vi "分析光源均勻度.vi"(7 "ShowData":bool, 8 "error in (no error)":errorcluster, 10 "DieArea":i32 min=10, 11 "Image In":T1) -> (0 "error out":errorcluster, 3 "Image":T1)   [LabVIEW 2015]
uses:
  <vilib>/vision/Image Controls.llb/IMAQ Image.ctl
  <vilib>/vision/NI_Vision_Development_Module.lvlib
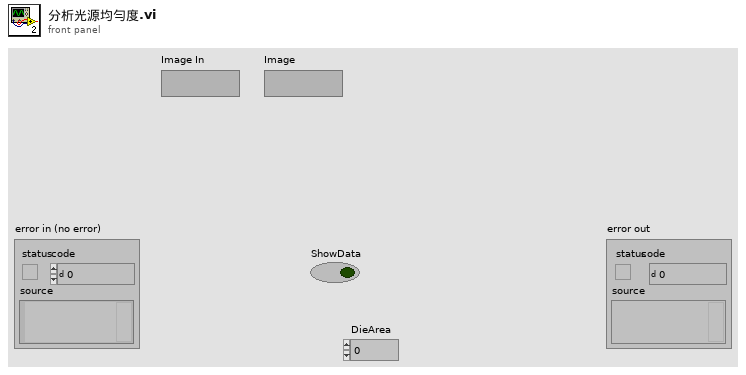
[diagram p1: front panel]
types:
  T1 = typedef "IMAQ Image.ctl" = refnum<image>
  T2 = cluster{"Left":i32, "Top":i32, "Right":i32, "Bottom":i32}
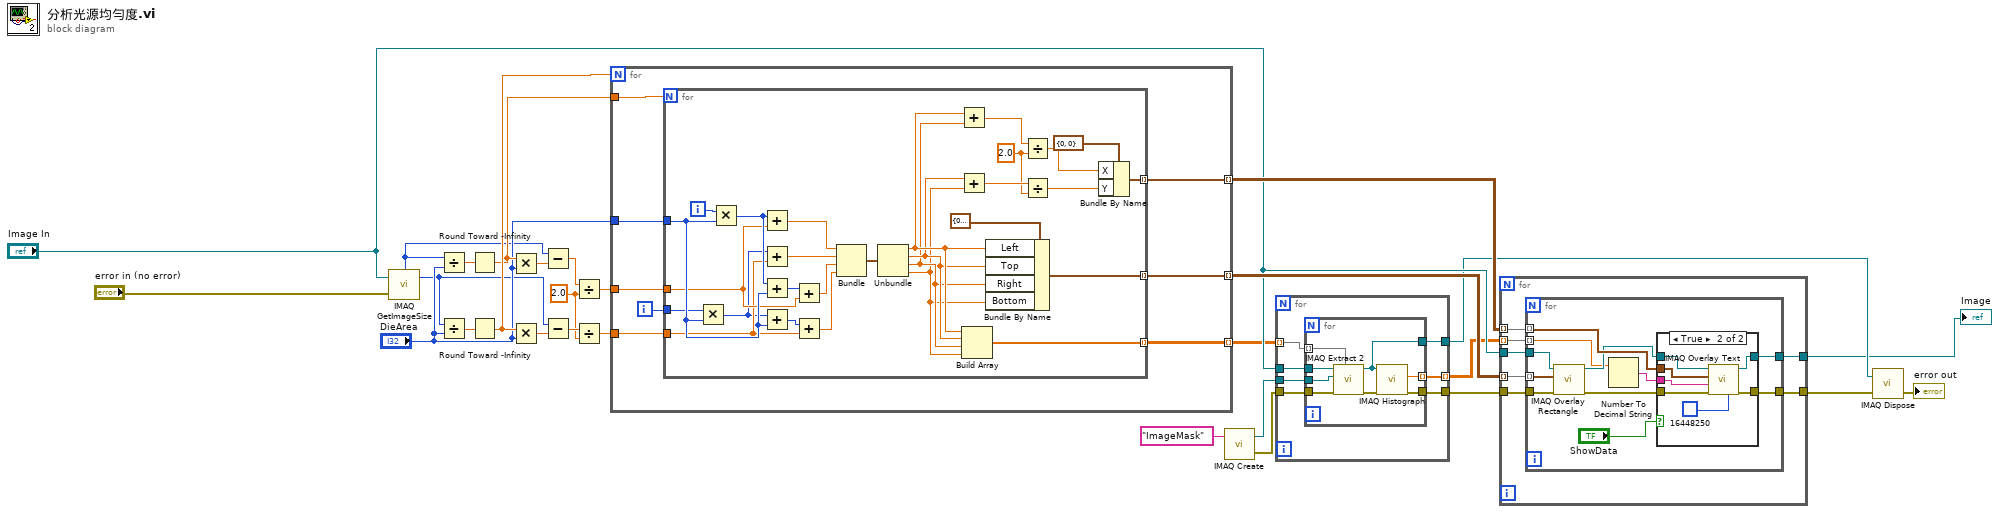
[diagram p0: block diagram]
diagram:
  w6 = 2.0 ("y")
  n1 = call "IMAQ GetImageSize"("Image"="Image In", "error in (no error)"="error in (no error)") -> ("Y Resolution"=w11:i32, "X Resolution"=w5:i32)  [unwired: 2 in, 1 out]
  n2 = Divide(x=w5, y="DieArea") -> (x/y=w28:dbl)
  n3 = Divide(x=w11, y="DieArea") -> (x/y=w27:dbl)
  n4 = Round Toward -Infinity(1:w28) -> (0:w13:dbl)
  n5 = Round Toward -Infinity(1:w27) -> (0:w14:dbl)
  n6 = Multiply(x=w13, y="DieArea") -> (x*y=w9:dbl)
  n7 = Multiply(x=w14, y="DieArea") -> (x*y=w10:dbl)
  n8 = Subtract(x=w5, y=w9) -> (x-y=w7:dbl)
  n9 = Subtract(x=w11, y=w10) -> (x-y=w8:dbl)
  n10 = Divide(x=w7, y=w6) -> (x/y=w4:dbl)
  n11 = Divide(x=w8, y=w6) -> (x/y=w3:dbl)
  n12 = for {
    N: w14 -> [_]
    tunnel: w13 -> [w36]
    tunnel: "DieArea" -> [w35]
    tunnel: [w34] -> w25 mode=indexing
    tunnel: [w33] -> w26 mode=indexing
    tunnel: [w32] -> w21 mode=indexing
    tunnel: w4 -> [w31]
    tunnel: w3 -> [w29]
    i -> [w30]
    n13 = for {
      N: w36 -> [_]
      tunnel: w30 -> [w62]
      tunnel: w35 -> [w64]
      tunnel: [w60] -> w34 mode=indexing
      tunnel: [w59] -> w33 mode=indexing
      tunnel: [w58] -> w32 mode=indexing
      tunnel: w31 -> [w44]
      tunnel: w29 -> [w41]
      i -> [w52]
      w55 = 2.0 ("y")
      n14 = Multiply(x=w62, y=w64) -> (x*y=w40:i32)
      n15 = Multiply(x=w52, y=w64) -> (x*y=w46:i32)
      n16 = Add(x=w46, y=w44) -> (x+y=w45:dbl)
      n17 = Add(x=w40, y=w41) -> (x+y=w39:dbl)
      n18 = Add(x=w46, y=w64) -> (x+y=w43:i32)
      n19 = Add(x=w40, y=w64) -> (x+y=w38:i32)
      n20 = Add(x=w43, y=w44) -> (x+y=w42:dbl)
      n21 = Add(x=w38, y=w41) -> (x+y=w37:dbl)
      n22 = Bundle(w45, w39, w42, w37) -> (w51:cluster{dbl, dbl, dbl, dbl})  [unwired: 1 in]
      n23 = Unbundle(w51) -> (w50:dbl, w49:dbl, w48:dbl, w47:dbl)
      n24 = Add(x=w50, y=w48) -> (x+y=w56:dbl)
      n25 = Add(x=w49, y=w47) -> (x+y=w57:dbl)
      n26 = Build Array(w50, w49, w48, w47) -> (w58:dbl[])
      n27 = Bundle By Name(cluster=T2 {"Left"=0, "Top"=0, "Right"=0, "Bottom"=0} ("Rectangle"), "Left"=w50, "Top"=w49, "Right"=w48, "Bottom"=w47) -> (w60:T2)
      n28 = Divide(x=w56, y=w55) -> (x/y=w53:dbl)
      n29 = Divide(x=w57, y=w55) -> (x/y=w54:dbl)
      n30 = Bundle By Name(cluster=cluster{"X":i32, "Y":i32} {"X"=0, "Y"=0} ("Origin"), "X"=w53, "Y"=w54) -> (w59:cluster{"X":i32, "Y":i32})
    }
  }
  n31 = call "IMAQ Create"("Image Name"="ImageMask") -> ("New Image"=w22:T1, "error out"=w19:errorcluster)  [unwired: 4 in]
  n32 = for {
    tunnel: "Image In" -> [w71]
    tunnel: w22 -> [w70]
    tunnel: w21 -> [w69] mode=indexing
    tunnel: [w68] -> w20 mode=indexing
    tunnel: w19 -> [w67]
    tunnel: [w66] -> w18
    tunnel: [w65] -> w2
    n33 = for {
      tunnel: w71 -> [w77]
      tunnel: w70 -> [w78]
      tunnel: w69 -> [w79] mode=indexing
      tunnel: [w76] -> w68 mode=indexing
      tunnel: w67 -> [w75]
      tunnel: [w73] -> w66
      tunnel: [w72] -> w65
      n34 = call "IMAQ Extract 2"("Optional Rectangle"=w79, "error in (no error)"=w75, "Image Dst"=w78, "Image Src"=w77) -> ("error out"=w74:errorcluster, "Image Dst Out"=w72:T1)  [unwired: 6 in]
      n35 = call "IMAQ Histograph"("error in (no error)"=w74, "Image"=w72) -> ("error out"=w73:errorcluster, "Mean Value"=w76:sgl)  [unwired: 6 in, 2 out]
    }
  }
  n36 = for {
    tunnel: w26 -> [w86] mode=indexing
    tunnel: w25 -> [w85] mode=indexing
    tunnel: "Image In" -> [w84]
    tunnel: [w83] -> w1
    tunnel: w20 -> [w82] mode=indexing
    tunnel: w18 -> [w81]
    tunnel: [w80] -> w17
    n37 = for {
      tunnel: w86 -> [w97] mode=indexing
      tunnel: w85 -> [w96] mode=indexing
      tunnel: w84 -> [w95]
      tunnel: [w93] -> w83
      tunnel: w82 -> [w92] mode=indexing
      tunnel: w81 -> [w90]
      tunnel: [w88] -> w80
      n38 = call "IMAQ Overlay Rectangle"("error in (no error)"=w90, "Rectangle"=w96, "Image"=w95) -> ("error out"=w89:errorcluster, "Image Out"=w94:T1)  [unwired: 7 in]
      n39 = Number To Decimal String(number=w92) -> (decimal integer string=w91:string)  [unwired: 1 in]
      n40 = case shown="True" "ShowData" {
        tunnel: w97 -> [_ w106]
        tunnel: w94 -> [w98 w105]
        tunnel: [w98 w104] -> w93
        tunnel: w91 -> [_ w103]
        tunnel: w89 -> [w99 w102]
        tunnel: [w99 w101] -> w88
        frame False {
        }
        frame True {
          n41 = call "IMAQ Overlay Text"("BG Color (Transparent)"=u32 16448250, "error in (no error)"=w102, "String"=w103, "Origin"=w106, "Image"=w105) -> ("error out"=w101:errorcluster, "Image Out"=w104:T1)  [unwired: 5 in]
        }
      }
    }
  }
  "Image" <- w1
  n42 = call "IMAQ Dispose"("Image"=w2, "error in (no error)"=w17) -> ("error out"=→"error out":errorcluster)  [unwired: 4 in]
